vi "from_string.vi"(8 "error in (no error)":errorcluster, 10 "string":string) -> (0 "error out":errorcluster, 3 "Item out":refnum<class "Item.lvclass">)   [LabVIEW 2020, in "toml_edit.lvlib" / "Item.lvclass"]
uses:
  Item.lvclass
  Item.lvclass/Item.ctl
  dragon_toml_64.dll
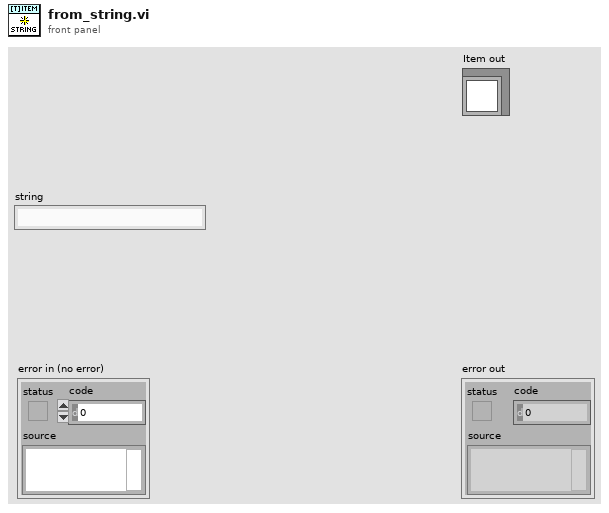
[diagram p1: front panel]
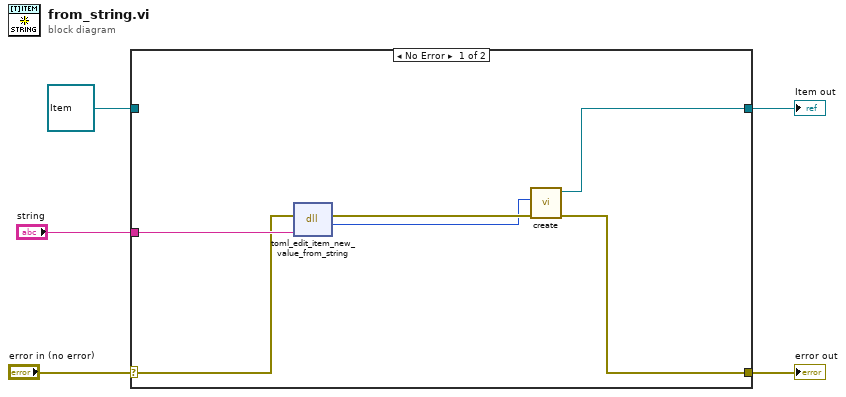
[diagram p0: block diagram]
diagram:
  n1 = case shown="No Error" "error in (no error)" {
    selector: "error in (no error)" -> [w7 w13]
    tunnel: [w6 w13] -> w4
    tunnel: [w11 w12] -> w2
    tunnel: refnum<class "Item.lvclass"> refnum ("Item in") -> [_ w12]
    tunnel: "string" -> [w10 _]
    frame No Error {
      n2 = dll-call lib="C:/Users/JamesMcNally/Documents/toml-edit-labview/lv_src/dragon_toml_*.*" fn="toml_edit_item_new_value_from_string"(error in=w7, "toml_string"=w10) -> (error out=w9:errorcluster, "doc_ref"=w8:u64)  [unwired: 3 in, 1 out]
      n3 = call "create.vi"("error in (no error)"=w9, "ref"=w8) -> ("error out"=w6:errorcluster, "Item out"=w11:refnum<class "Item.lvclass">)  [unwired: 7 in, 1 out]
    }
    frame Error {
    }
  }
  "error out" <- w4
  "Item out" <- w2
